vi "CPU_MEM_RAM_WR.vi"(10 "value in":u8 format="%02x", 11 "address":u16 format="%.0x") -> ()   [LabVIEW 2018]
uses:
  CPU_MEM_references.vi
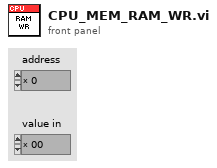
[diagram p1: front panel]
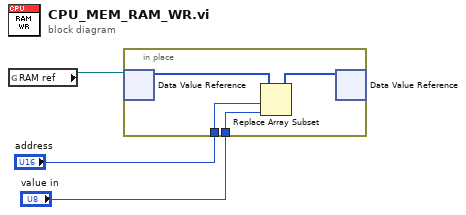
[diagram p0: block diagram]
diagram:
  n1 = global read "CPU_MEM_references.vi" "RAM ref"() -> (w1:refnum<data-value>)
  n2 = in-place {
    in-place-border: "value in" -> [w7]
    in-place-border: "address" -> [w6]
    n3 = in-place-dvr #1(w1) -> (w5:u8[])  [unwired: 1 out]
    n4 = Replace Array Subset(array=w5, new element=w7, index=w6) -> (w4:u8[])
    n5 = in-place-dvr #1(w4) -> ()  [unwired: 2 out]
  }
